vi "MessageName.vi"() -> (2 "MessageName":string)   [LabVIEW 2020, in "Error.lvlib"]
uses:
  Error.lvlib
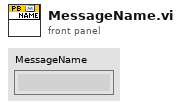
[diagram p1: front panel]
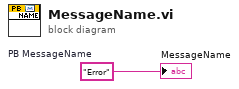
[diagram p0: block diagram]
diagram:
  w1 = "Error"  # PB MessageName
  "MessageName" <- w1
